vi "실습 8-4.vi"() -> ()   [LabVIEW 2014]
panel:
  in  "WebBrowser":refnum<k7>(container)
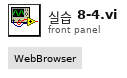
[diagram p1: front panel]
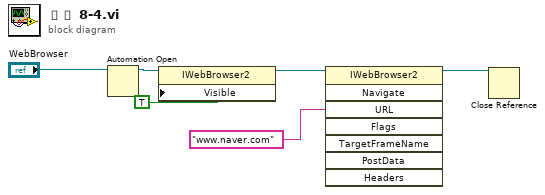
[diagram p0: block diagram]
diagram:
  n1 = Automation Open(Automation Refnum="WebBrowser") -> (Automation Refnum=w5:refnum<k7>)  [unwired: 3 in, 1 out]
  n2 = property class="IWebBrowser2"(reference=w5, "Visible"=TRUE) -> (reference out=w3:refnum<k7>)  [unwired: 1 in, 1 out]
  n3 = invoke class="IWebBrowser2" method="Navigate"(reference=w3, "URL"="www.naver.com") -> (reference out=w1:refnum<k7>)  [unwired: 6 in, 7 out]
  n4 = Close Reference(reference=w1) -> ()  [unwired: 1 in, 1 out]
